vi "Move Control Mouse LV2016 NIVerified.vi"() -> ()   [LabVIEW 2016]
uses:
  <vilib>/Utility/miscctls.llb/LVBoundsTypeDef.ctl
panel:
  in  "stop":bool
  out "Boolean":bool
  # "Overview:\nThis example is based on the following example:\nDrag and Drop Controls and Indicators on Front Panel (https://decibel.ni.com/content/docs/DOC-3577)\nThe difference is that this example moves the front panel control/indicator while the mouse is moving and not after the mouse button has been released.\nRequirements:\nLabVIEW 8.0 (or compatible)\nInstructions:\nTo run this example, simply run the VI and click on the Boolean control and move the mouse."
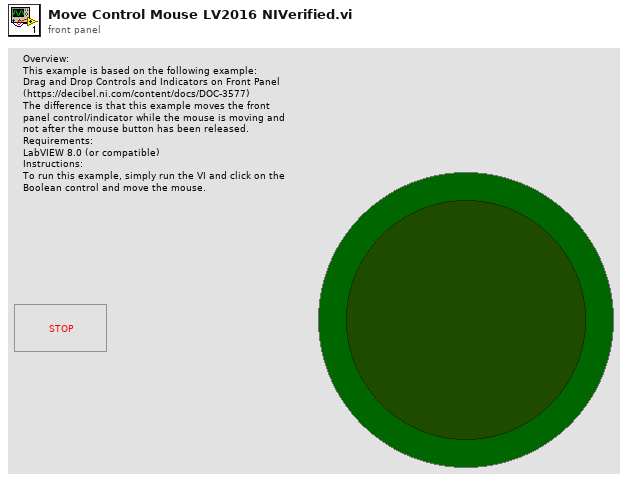
[diagram p1: front panel]
types:
  T1 = typedef "LVBoundsTypeDef.ctl" = cluster{"Width":u32, "Height":u32}
  T2 = typedef "LVPoint32TypeDef.ctl" = cluster{"Horizontal":i32, "Vertical":i32}
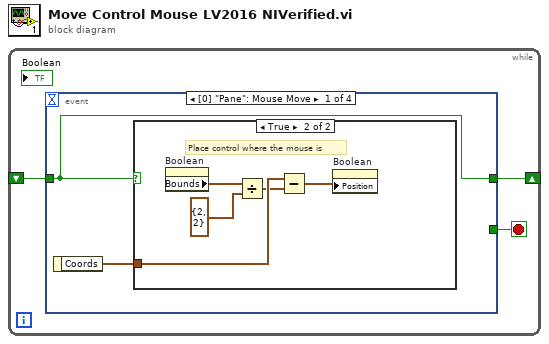
[diagram p0: block diagram]
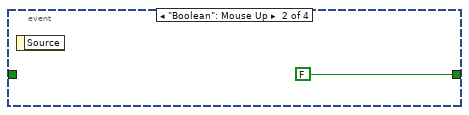
[diagram p3: hidden frame]
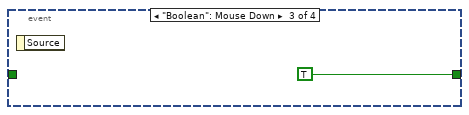
[diagram p4: hidden frame]
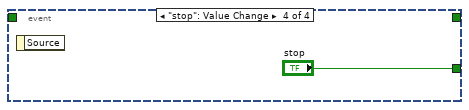
[diagram p5: hidden frame]
diagram:
  n1 = while {
    shift-right: [w2] -> _
    shift-left: _ -> [w1]
    stop <- w3 stop-if-true
    n2 = event shown="[0] \"Pane\": Mouse Move" {
      selector: _ -> [_ _ _ _]
      dyn-events: _ -> [_ _ _ _]
      timeout: _ -> [_ _ _ _]
      tunnel: [_ _ _ "stop"] -> w3
      tunnel: [w4 FALSE TRUE _] -> w2
      tunnel: w1 -> [w4 _ _ _]
      event Mouse Move {
        n3 = event-data() -> ("Coords"=w5:T2)  [unwired: 1 out]
        n4 = case shown="True" w4 {
          tunnel: w5 -> [_ w7]
          frame False {
          }
          frame True {
            # "Place control where the mouse is"
            n5 = property on="Boolean" class="Bool (strict)"() -> ("Bounds"=w10:T1)  [unwired: 2 in, 2 out]
            n6 = Divide(x=w10, y=T1 {"Width"=2, "Height"=2}) -> (x/y=w6:cluster{"Width":dbl, "Height":dbl})
            n7 = Subtract(x=w7, y=w6) -> (x-y=w8:cluster{dbl, dbl})
            n8 = property on="Boolean" class="Bool (strict)"("Position"=w8) -> ()  [unwired: 2 in, 2 out]
          }
        }
      }
      event "Boolean": Mouse Up {
        n9 = event-data() -> ()  [unwired: 2 out]
      }
      event "Boolean": Mouse Down {
        n10 = event-data() -> ()  [unwired: 2 out]
      }
      event "stop": Value Change {
        n11 = event-data() -> ()  [unwired: 2 out]
      }
    }
  }
